vi "CHECK TIME.vi"(11 "EMAILS SENT IN":bool=TRUE) -> (2 "SEND EMAILS?":bool=TRUE, 3 "EMAILS SENT OUT":bool=TRUE)   [LabVIEW 2019]
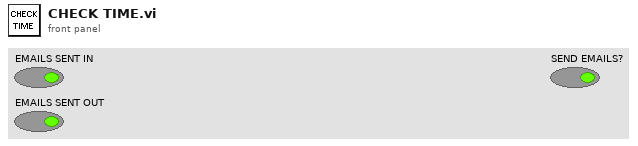
[diagram p1: front panel]
types:
  T1 = typedef "LVDateTimeRec.ctl" = cluster{"fractional second":dbl, "second":i32, "minute":i32, "hour":i32, "day of month":i32, "month":i32, "year":i32, "day of week":i32, "day of year":i32, "DST":i32}
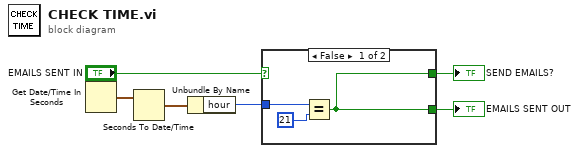
[diagram p0: block diagram]
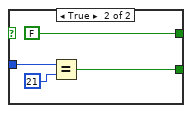
[diagram p2: hidden frame]
diagram:
  n1 = Get Date/Time In Seconds() -> (seconds since 1Jan1904=w6:timestamp)
  n2 = Seconds To Date/Time(time stamp (now)=w6) -> (date time rec=w5:T1)  [unwired: 1 in]
  n3 = Unbundle By Name(w5) -> ("hour"=w3:i32)
  n4 = case shown="False" "EMAILS SENT IN" {
    tunnel: w3 -> [w9 w13]
    tunnel: [w7 w11] -> w2
    tunnel: [w7 FALSE] -> w1
    frame False {
      n5 = Equal?(x=w9, y=21) -> (x = y?=w7:bool)
    }
    frame True {
      n6 = Equal?(x=w13, y=21) -> (x = y?=w11:bool)
    }
  }
  "EMAILS SENT OUT" <- w2
  "SEND EMAILS?" <- w1
